vi "Wiggle Node to Grab Wire.vi"(8 "error in (no error)":errorcluster, 10 "Wiggle Size (px)":i32, 11 "Node in":refnum<vi>) -> (0 "error out":errorcluster, 3 "Node out":refnum<vi>)   [LabVIEW 2020, in "JKI State Machine API.lvlib" / "JKI SM.lvclass"]
uses:
  JKI SM.lvclass
  JKI SM.lvclass/JKI SM.ctl
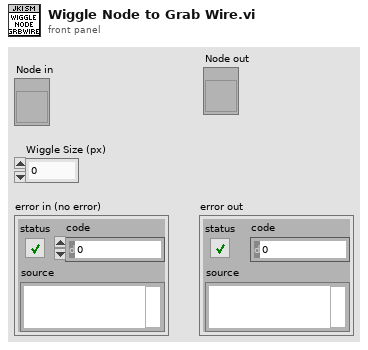
[diagram p1: front panel]
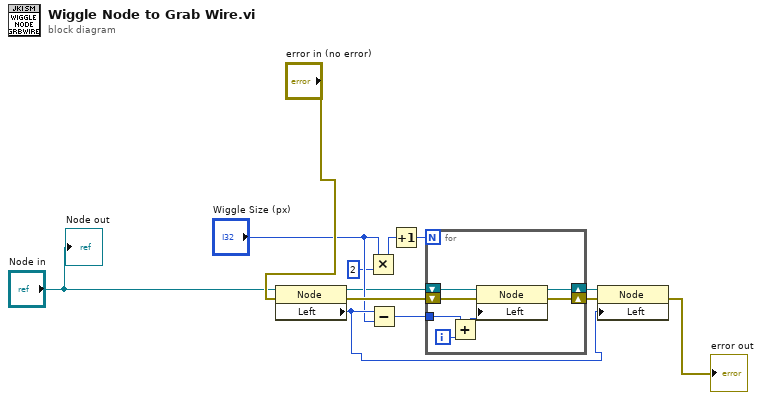
[diagram p0: block diagram]
diagram:
  n1 = property class="Node"(reference="Node in", error in="error in (no error)") -> (reference out=w2:refnum<vi>, error out=w11:errorcluster, "Left"=w9:i32)
  n2 = Multiply(x="Wiggle Size (px)", y=2) -> (x*y=w3:i32)
  n3 = Subtract(x=w9, y="Wiggle Size (px)") -> (x-y=w7:i32)
  n4 = Increment(x=w3) -> (x+1=w4:i32)
  n5 = for {
    N: w4 -> [_]
    shift-right: [w18] -> w8
    shift-left: w2 -> [w17]
    tunnel: w7 -> [w19]
    shift-right: [w15] -> w10
    shift-left: w11 -> [w14]
    i -> [w20]
    n6 = Add(x=w19, y=w20) -> (x+y=w16:i32)
    n7 = property class="Node"(reference=w17, error in=w14, "Left"=w16) -> (reference out=w18:refnum<vi>, error out=w15:errorcluster)
  }
  n8 = property class="Node"(reference=w8, error in=w10, "Left"=w9) -> (error out=→"error out":errorcluster)  [unwired: 1 out]
  "Node out" <- "Node in"
